vi "Stop.vi"(8 "Error In":errorcluster, 11 "reference in":refnum<class "Camera.lvclass">) -> (0 "Error Out":errorcluster, 3 "reference out":refnum<class "Camera.lvclass">)   [LabVIEW 2025, in "Camera.lvclass"]
uses:
  Camera.lvclass
  Interfaces/IRunnable/IRunnable.lvclass
  <vilib>/ActorFramework/Message Enqueuer/Message Enqueuer.lvclass/Message Enqueuer.ctl
  <vilib>/ActorFramework/Message Enqueuer/Enqueue.vi
  <vilib>/ActorFramework/Stop Msg/Stop Msg.lvclass
  <vilib>/ActorFramework/Message Priority Queue/Priority Enqueue.vi
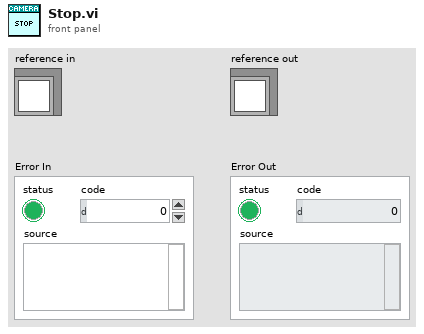
[diagram p1: front panel]
types:
  T1 = typedef "Camera.lvclass/ObjectAttributes.ctl" = cluster{"IConfigure":refnum<class "IConfigure.lvclass">, "Worker Enqueuer":refnum<class "Message Enqueuer.lvclass">, "Start Counter":i32, "Initialized":bool}
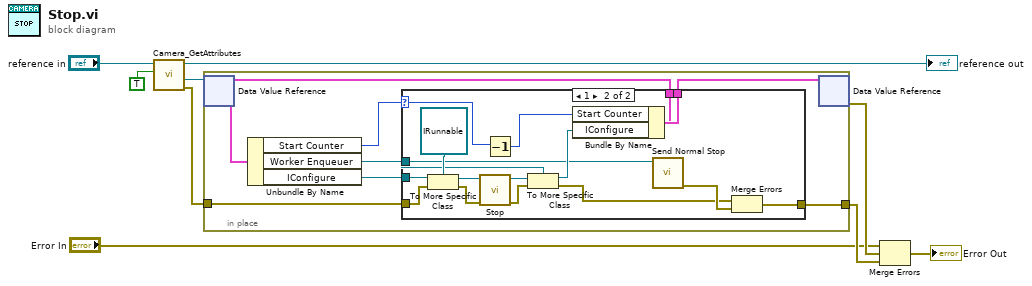
[diagram p0: block diagram]
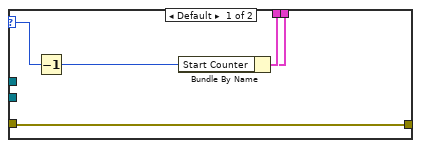
[diagram p2: hidden frame]
diagram:
  n1 = call "Camera_GetAttributes.vi"("OnlyGetDvrReference(False)"=TRUE, "reference in"="reference in") -> ("Error Out"=w4:errorcluster, "DataRef"=w5:refnum<data-value>, "reference out"=→"reference out":refnum<class "Camera.lvclass">)  [unwired: 6 in, 1 out]
  n2 = in-place {
    in-place-border: [w11] -> w9
    in-place-border: w4 -> [w13]
    n3 = in-place-dvr #1(w5) -> (w15:T1)  [unwired: 1 out]
    n4 = Unbundle By Name(w15) -> ("Start Counter"=w10:i32, "Worker Enqueuer"=w12:refnum<class "Message Enqueuer.lvclass">, "IConfigure"=w14:refnum<class "IConfigure.lvclass">)
    n5 = case shown="1" w10 {
      selector: w10 -> [w21 w26]
      tunnel: [w19 w37] -> w16
      tunnel: w15 -> [w20 w36]
      tunnel: w14 -> [_ w29]
      tunnel: w13 -> [w17 w28]
      tunnel: w12 -> [_ w27]
      tunnel: [w17 w24] -> w11
      frame Default {
        n6 = Decrement(x=w21) -> (x-1=w18:i32)
        n7 = Bundle By Name(cluster=w20, "Start Counter"=w18) -> (w19:T1)
      }
      frame 1 {
        n8 = To More Specific Class(target class=refnum<class "IRunnable.lvclass"> refnum ("IRunnable.lvclass"), reference=w29, error in=w28) -> (specific class reference=w32:refnum<class "IRunnable.lvclass">, error out=w33:errorcluster)
        n9 = call-dynamic "Stop.vi"("error in"=w33, "IRunnable in"=w32) -> ("error out"=w31:errorcluster, "IRunnable out"=w30:refnum<class "IRunnable.lvclass">)  [unwired: 8 in]
        n10 = Decrement(x=w26) -> (x-1=w25:i32)
        n11 = To More Specific Class(target class=w29, reference=w30, error in=w31) -> (specific class reference=w34:refnum<class "IConfigure.lvclass">, error out=w22:errorcluster)
        n12 = Bundle By Name(cluster=w36, "Start Counter"=w25, "IConfigure"=w34) -> (w37:T1)
        n13 = call <vilib>:"Send Normal Stop.vi"("Message Enqueuer"=w27) -> ("error out"=w23:errorcluster)  [unwired: 10 in]
        n14 = Merge Errors(w22, w23) -> (w24:errorcluster)
      }
    }
    n15 = in-place-dvr #1(w16) -> (w2:errorcluster)  [unwired: 1 out]
  }
  n16 = Merge Errors("Error In", w2, w9) -> (→"Error Out":errorcluster)
